vi "单向画图.vi"(1 "电流数据":dbl[](array[numeric]), 2 "电压改变量":dbl, 4 "电压范围":dbl) -> (0 "XY图":picture)   [LabVIEW 2019]
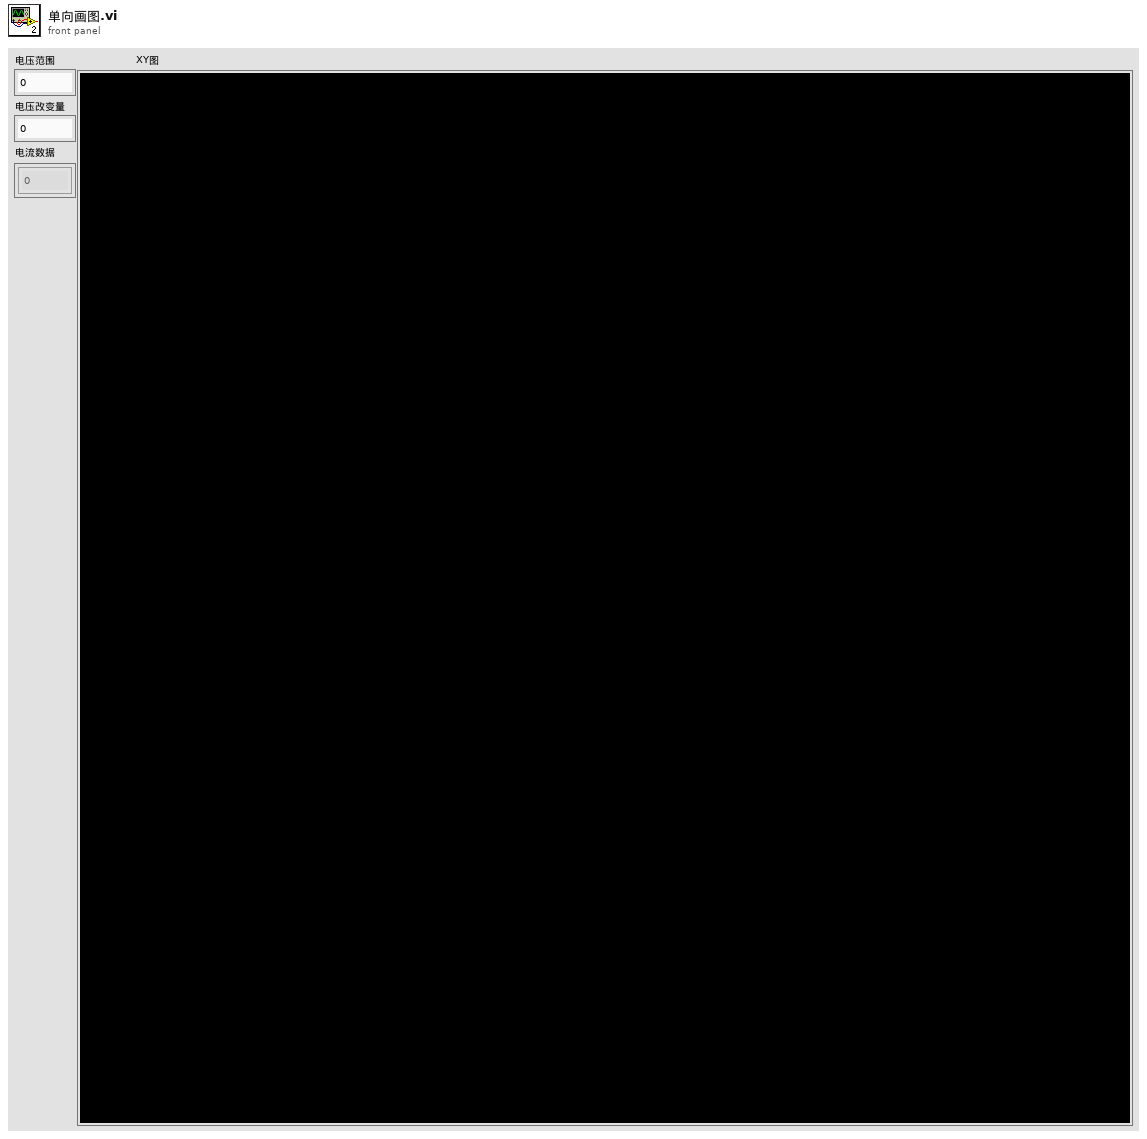
[diagram p1: front panel]
types:
  T1 = enum8{"Decimal", "Scientific", "Engineering", "Binary", "Octal", "Hex"}
  T2 = cluster{dbl, dbl, "x log?":bool, "x precision":u8, "x format":enum8{"Decimal", "Scientific", "Engineering", "Binary", "Octal", "Hex"}, dbl, dbl, "y log?":bool, "y precision":u8, "y format":enum8{"Decimal", "Scientific", "Engineering", "Binary", "Octal", "Hex"}}
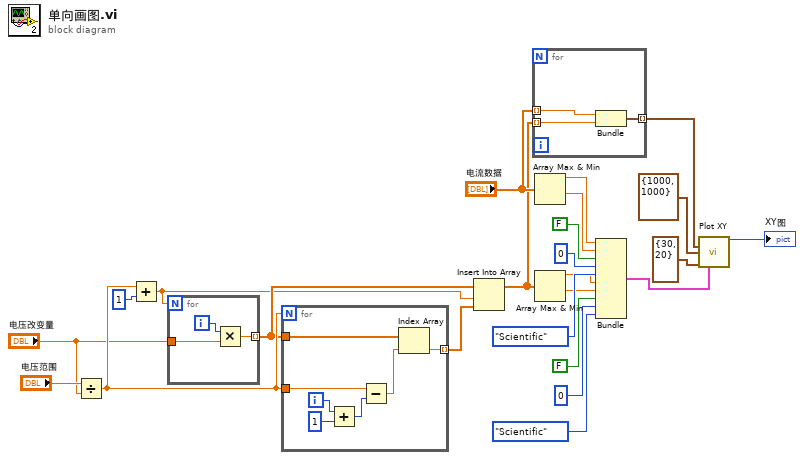
[diagram p0: block diagram]
diagram:
  n1 = Divide(x="电压范围", y="电压改变量") -> (x/y=w7:dbl)
  n2 = Add(x=w7, y=1) -> (x+y=w4:dbl)
  n3 = for {
    N: w4 -> [_]
    tunnel: "电压改变量" -> [w27]
    tunnel: [w26] -> w6 mode=indexing
    i -> [w25]
    n4 = Multiply(x=w25, y=w27) -> (x*y=w26:dbl)
  }
  n5 = for {
    N: w7 -> [_]
    tunnel: w6 -> [w34]
    tunnel: w7 -> [w33]
    tunnel: [w31] -> w5 mode=indexing
    i -> [w30]
    n6 = Add(x=w30, y=1) -> (x+y=w28:i32)
    n7 = Subtract(x=w33, y=w28) -> (x-y=w32:dbl)
    n8 = Index Array(array=w34, index=w32) -> (element=w31:dbl)
  }
  n9 = Insert Into Array(array=w6, index=w4, new element=w5) -> (w2:dbl[])
  n10 = for {
    tunnel: [w37] -> w24 mode=indexing
    tunnel: "电流数据" -> [w36] mode=indexing
    tunnel: w2 -> [w35] mode=indexing
    n11 = Bundle("数值"=w36, w35) -> (w37:cluster{"数值":dbl, dbl})  [unwired: 1 in]
  }
  n12 = Array Max & Min(array="电流数据") -> (max value=w9:dbl, min value=w8:dbl)  [unwired: 2 out]
  n13 = Array Max & Min(array=w2) -> (max value=w12:dbl, min value=w11:dbl)  [unwired: 2 out]
  n14 = Bundle(w9, w8, "x log?"=FALSE, "x precision"=u8 0, "x format"=T1."Scientific", w12, w11, "y log?"=FALSE, "y precision"=u8 0, "y format"=T1."Scientific") -> (w16:T2)  [unwired: 1 in]
  n15 = call <vilib>:"Plot XY.vi"("data"=w24, "dimensions (w,h)"=cluster{"width":i16, "height":i16} {"width"=1000, "height"=1000}, "top left point(0, 0)"=cluster{"x":i16, "y":i16} {"x"=30, "y"=20}, "cartesian axis attributes"=w16) -> ("new picture"=→"XY图":picture)  [unwired: 11 in]
